vi "Error 5032.vi"(8 "error in (no error)":errorcluster, 10 "Path":path) -> (0 "error out":errorcluster)   [LabVIEW 2019, in "gRPC Template Creation Utility.lvlib"]
uses:
  gRPC Template Creation Utility.lvlib
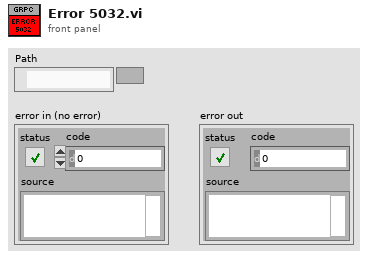
[diagram p1: front panel]
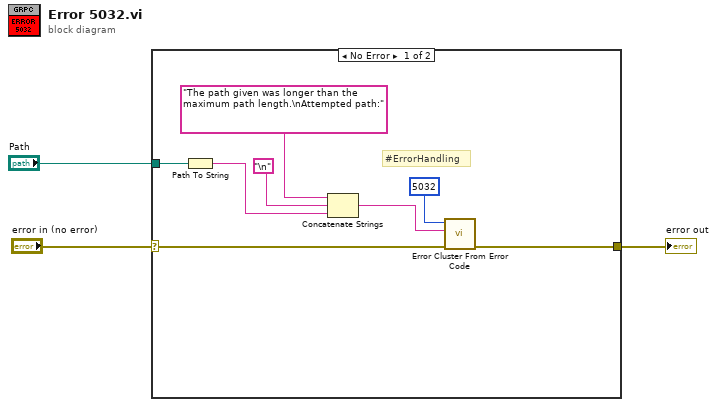
[diagram p0: block diagram]
diagram:
  n1 = case shown="No Error" "error in (no error)" {
    selector: "error in (no error)" -> [w5 w12]
    tunnel: [w11 w12] -> w3
    tunnel: "Path" -> [w9 _]
    frame No Error {
      # "#ErrorHandling"
      n2 = Path To String(path=w9) -> (string=w4:string)
      n3 = Concatenate Strings("The path given was longer than the maximum path length.\nAttempted path:" ("error message (\"\")"), "\n", w4) -> (w10:string)
      n4 = call <vilib>:"Error Cluster From Error Code.vi"("error in (no error)"=w5, "error message (\"\")"=w10, "error code (0)"=5032) -> ("error out"=w11:errorcluster)  [unwired: 6 in]
    }
    frame Error {
    }
  }
  "error out" <- w3
